vi "XPS hardware acquire.vi"(8 "error in (no error)":errorcluster, 11 "Object in":refnum<class "NewportXPS.lvclass">) -> (0 "error out":errorcluster, 3 "Object out":refnum<class "NewportXPS.lvclass">)   [LabVIEW 2020, in "NewportXPS.lvclass"]
uses:
  NewportXPS.lvclass
  XPS Acquire FGV.ctl
  shared/stop FGV control.ctl
  NewportXPS.lvclass/NewportXPS.ctl
  BaseDriver/DriverMsg.ctl
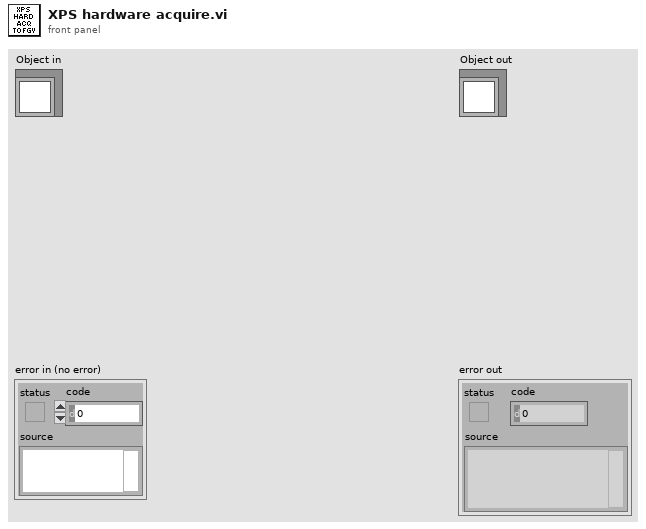
[diagram p1: front panel]
types:
  T1 = typedef "stop FGV control.ctl" = enum16{"Clear", "Write", "Read"}
  T2 = typedef "XPS Acquire FGV.ctl" = cluster{"busy":bool, "positions":dbl[], "PositionTable":variant}
  T3 = cluster{"Axis 1":string, "Axis 2":string, "Axis 3":string, "Axis 4":string, "Axis 5":string, "Axis 6":string}
  T4 = typedef "DriverMsg.ctl" = cluster{"Command":string, "Args":string[]}
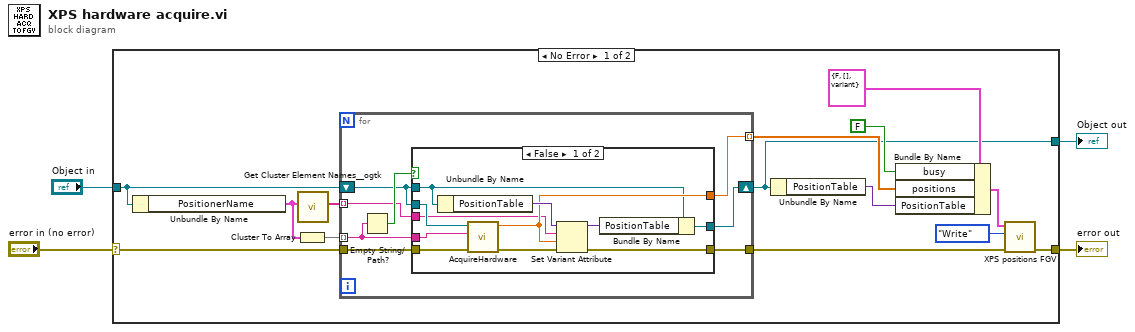
[diagram p0: block diagram]
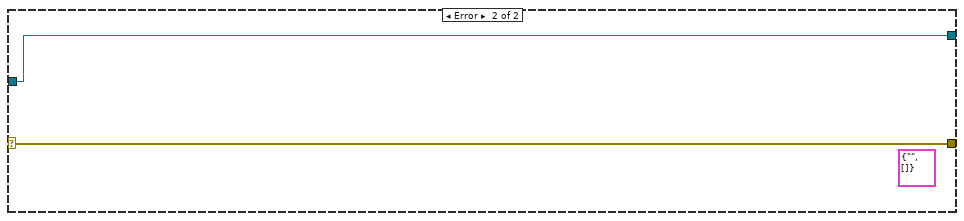
[diagram p3: hidden frame]
diagram:
  n1 = case shown="No Error" "error in (no error)" {
    selector: "error in (no error)" -> [w17 w41]
    tunnel: [w11 w41] -> w2
    tunnel: [w6 w40] -> w1
    tunnel: "Object in" -> [w9 w40]
    frame No Error {
      n2 = Unbundle By Name(w9) -> ("PositionerName"=w8:T3)
      n3 = Cluster To Array(cluster=w8) -> (array=w18:string[])
      n4 = call <userlib>:"Get Cluster Element Names__ogtk.vi"("Cluster"=w8) -> ("Element Names"=w7:string[])  [unwired: 9 in, 1 out]
      n5 = for {
        tunnel: [w26] -> w12
        tunnel: w18 -> [w24] mode=indexing
        tunnel: w17 -> [w25]
        tunnel: [w23] -> w14 mode=indexing
        shift-right: [w20] -> w6
        shift-left: w9 -> [w21]
        tunnel: w7 -> [w19] mode=indexing
        n6 = Empty String/Path?(string/path=w24) -> (empty?=w22:bool)
        n7 = case shown="False" w22 {
          tunnel: [w31 w39] -> w26
          tunnel: w25 -> [w37 w39]
          tunnel: w24 -> [w34 _]
          tunnel: [w33 _] -> w23
          tunnel: w21 -> [w36 _]
          tunnel: w21 -> [w30 w38]
          tunnel: [w28 w38] -> w20
          tunnel: w19 -> [w27 _]
          frame False {
            n8 = Unbundle By Name(w30) -> ("PositionTable"=w35:variant)
            n9 = call-dynamic "AcquireHardware.vi"("error in (no error)"=w37, "Axis 1"=w34, "NewportXPS in"=w36) -> ("error out"=w32:errorcluster, "Current position (units)"=w33:dbl)  [unwired: 7 in]
            n10 = Set Variant Attribute(Variant=w35, name=w27, value=w33, error in=w32) -> (Variant out=w29:variant, error out=w31:errorcluster)  [unwired: 1 out]
            n11 = Bundle By Name(cluster=w30, "PositionTable"=w29) -> (w28:refnum<class "NewportXPS.lvclass">)
          }
          frame True {
          }
        }
      }
      n12 = Unbundle By Name(w6) -> ("PositionTable"=w5:variant)
      n13 = Bundle By Name(cluster=T2 {"busy"=FALSE, "positions"=[], "PositionTable"=variant} ("Acq Data in"), "busy"=FALSE, "positions"=w14, "PositionTable"=w5) -> (w15:T2)
      n14 = call "XPS positions FGV.vi"("error in"=w12, "Function"=stop_FGV_control."Write", "Acq Data in"=w15) -> ("error out"=w11:errorcluster)  [unwired: 7 in, 1 out]
    }
    frame Error {
      (unwired) T4 {"Command"="", "Args"=[]} ("Msg out")
    }
  }
  "error out" <- w2
  "Object out" <- w1
